vi "NanotecSMCPD.halt axis.vi"(0 "i ref in":refnum<vi>, 1 "axis":i32, 2 "ManuelStop":bool, 3 "ms timeout (10000)":i32=10000, 5 "error in (no error)":errorcluster) -> (14 "i ref out":refnum<vi>, 17 "timed out":bool, 19 "error out":errorcluster)   [LabVIEW 2014, in "NanotecSMCPD.lvlib"]
doc: "Abruptly stops the ongoing movement of the specified axis, possible loss of steps."
uses:
  NanotecSMCPD.lvlib
  CSCore/CSSystem/CoreDefs/CoreDefs.error_type.ctl
  CSCore/CSSystem/CoreDefs/CoreDefs.error_severity.ctl
  CSCore/CSApplicationBaseClasses/MotorBase/MotorBase.statusType.ctl
  CSCore/CSApplicationBaseClasses/MotorBase/MotorBase.directionType.ctl
  CSCore/CSApplicationBaseClasses/MotorBase/MotorBase.serviceType.ctl
  CSlibraries/UtilityLib/UtilityLib.valueStatus.ctl
  CSCore/CSApplicationBaseClasses/DeviceBase/DeviceBase.lvlib
  CSCore/CSSystem/CoreLib/CoreLib.lvlib
  CSCore/CSApplicationBaseClasses/MotorBase/MotorBase.lvlib
  CSlibraries/UtilityLib/UtilityLib.lvlib
  CSinstr.lib/NanotecSMCPD/NanotecSMCPDDriver.lvlib
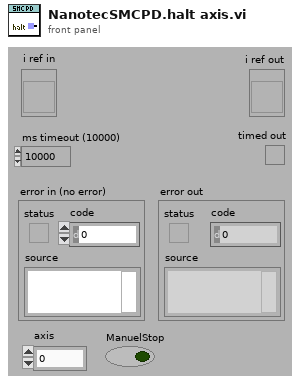
[diagram p1: front panel]
types:
  T1 = typedef "CoreDefs.error_severity.ctl" = enum16{"undefined", "information", "warning", "error", "fatal"}
  T2 = typedef "CoreDefs.error_type.ctl" = enum16{"no error", "can't load process", "can't unload process", "process does not exist", "can't install process", "can't remove process", "unknown function", "time out", "can't execute function", "duplicate queue name", "super not found", "caller queue invalid", "can't ping process", "unknown error", "VISA Error", "VISA timeout", "GPIB timeout", "GPIB error", "communication error", "data type mismatch", "can't read data from OPC server", "can't write data to OPC server", "OET error", "function not implemented", "process already exists", "invalid Shared Variable name", "error writing Shared Variable", "error reading Shared Variable", "invalid client name", "corrupt database", "unknown class", "call not authorized", "parameter out of range", "OET timeout: can't get data to modify", "invalid queue name", "requested operation incompatible with current state", "event undefined", "event disabled", "state undefined", "caller is not a friend", "EventBuilder: bad eventID", "EventBuilder: no DAQ devices", "a thread must not stop itself", "UNUSED ELEMENT4", "DiscArchiver: eventData incomplete", "DiscArchiver: eventData does not belong to run", "DiscArchiver: can't open file", "DiscArchiver: can't write to file", "DiscArchiver: available disc space low", "can't acquire semaphore", "error reading data from database", "notifier object is not existing", "can't register process", "can't unregister process", "illegal event type", "object disabled", "object already exists", "can't change state", "Instrument not found", "no connection to remote node", "invalid reference", "N/A", "UNUSED ELEMENT 1", "element not found", "illegal TCP/IP connection detected", "object does not exist", "invalid access ID", "unknown CS system", "invalid privilige", "unsupported data type", "unsupported server type", "IO server already exists", "Shared Variable already exists"}
  T3 = typedef "MotorBase.lvlib/MotorBase.serviceType.ctl" = enum16{"onOff", "startVelocity", "stopVelocity", "acceleration", "rangeMin", "rangeMax", "status", "position"}
  T4 = typedef "MotorBase.lvlib/MotorBase.directionType.ctl" = enum16{"unknown", "update actual value", "update nominal value", "update both"}
  T5 = typedef "UtilityLib.lvlib/UtilityLib.valueStatus.ctl" = enum16{"no info available", "stand by/off", "on", "warning", "alarm/malfunction", "not implemented", "user action required", "important information", "system default", "control default", "indicator default", "button default"}
  T6 = typedef "MotorBase.lvlib/MotorBase.statusType.ctl" = u32
  T7 = typedef "NanotecSMCPD.lvlib/NanotecSMCPD.i attribute.ctl" = cluster{"referencing":bool[], "stop":bool[], "AutoHalt ID":i32, "MethodQueue":refnum<queue>, "Referenced1Time?":bool[], "LastCommand ID":i32}
  T8 = typedef "MotorBase.lvlib/MotorBase.i attribute.ctl" = cluster{"defaultAxisIndex":i32, "logicalName":string[], "nOfAxes":i32, "physicalName":string[], "scaling":dbl[], "units":string[], "defaulAxisIndexID":i32, "logicalNameID":i32, "nOfAxesID":i32, "physicalNameID":i32, "unitID":i32, "actValues":T9, "nomValues":T9}
  T9 = typedef "MotorBase.lvlib/MotorBase.parameters.ctl" = cluster{"services":cluster{"onOff":bool[], "startVelocity":dbl[], "stopVelocity":dbl[], "acceleration":dbl[], "rangeMin":dbl[], "rangeMax":dbl[], "status":T6[], "position":dbl[]}, "serviceIDs":cluster{"onOffID":i32, "startVelocityID":i32, "stopVelocityID":i32, "accelerationID":i32, "rangeMinID":i32, "rangeMaxID":i32, "statusID":i32, "positionID":i32}}
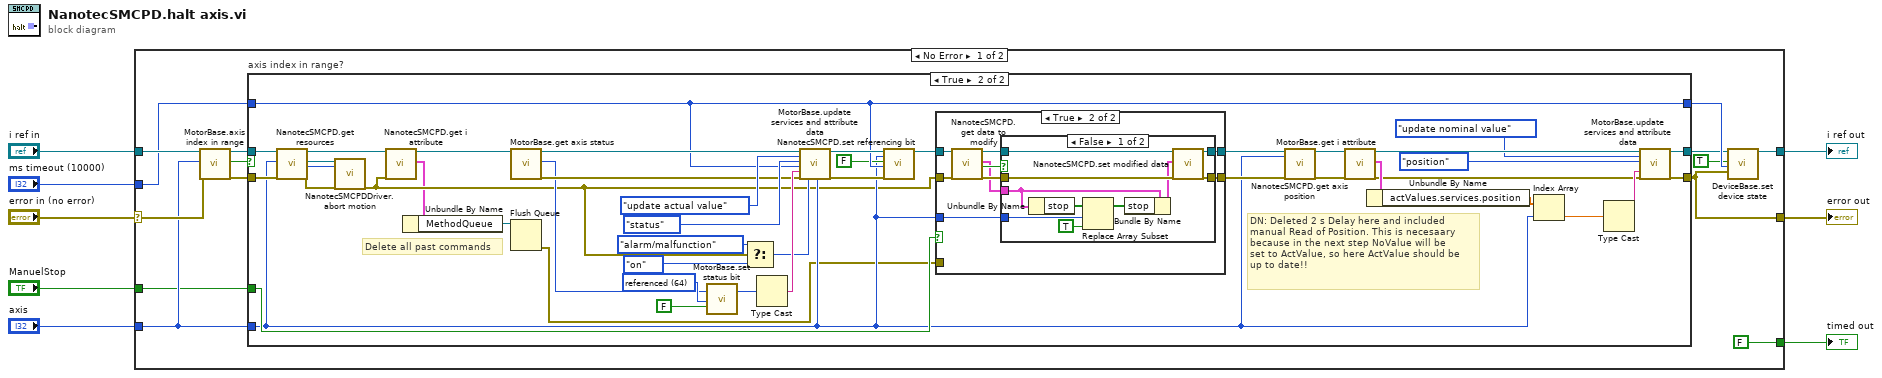
[diagram p0: block diagram]
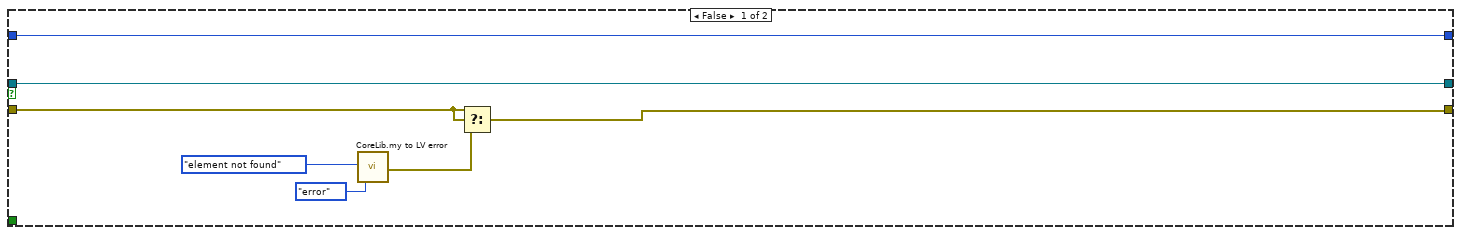
[diagram p2: hidden frame]
diagram:
  n1 = case shown="No Error" "error in (no error)" {
    selector: "error in (no error)" -> [w15 w97]
    tunnel: "ms timeout (10000)" -> [w12 _]
    tunnel: "i ref in" -> [w16 w98]
    tunnel: [w14 w97] -> w5
    tunnel: "axis" -> [w13 _]
    tunnel: [w11 w98] -> w3
    tunnel: [FALSE _] -> w2
    tunnel: "ManuelStop" -> [w9 _]
    frame No Error {
      n2 = call "MotorBase.axis index in range.vi"("i ref in"=w16, "axisIndex"=w13, "error in (no error)"=w15) -> ("i ref out"=w20:refnum<vi>, "in range"=w19:bool, "error out"=w21:errorcluster)  [unwired: 14 in]
      n3 = case "axis index in range?" shown="True" w19 {
        tunnel: [w29 w41] -> w18
        tunnel: [w26 w42] -> w14
        tunnel: w12 -> [w23 w54]
        tunnel: w13 -> [_ w36]
        tunnel: w20 -> [w29 w68]
        tunnel: w21 -> [w27 w67]
        tunnel: [w23 w54] -> w22
        tunnel: w9 -> [_ w52]
        frame False {
          n4 = call "CoreLib.my to LV error.vi"("ErrorTypes"=CoreDefs.error_type."element not found", "severityLevel"=CoreDefs.error_severity."error") -> ("myErrorCluster"=w25:errorcluster)  [unwired: 16 in, 1 out]
          n5 = Select(t=w27, s=w27, f=w25) -> (s? t:f=w26:errorcluster)
        }
        frame True {
          w64 = T6 64 items=["motorEnabled"=1, "negativeLimitSwitchActive"=2, "positiveLimitSwitchActive"=4, "limitSwitchesEnabled"=8, "limitSwitchesAreNormallyClosed"=16, "reseved1"=32, "referenced"=64, "inPosition"=128, "reserved2"=256, "reserved3"=512, "reserved4"=1024, "reserved5"=2048, "error"=4096, "reserved6"=8192, "reserved7"=16384, "reserved8"=32768, "user defined1"=65536, "user defined2"=131072, "user defined3"=262144, "user defined4"=524288, "user defined5"=1048576, "user defined6"=2097152, "user defined7"=4194304, "user defined8"=8388608, "user defined9"=16777216, "user defined10"=33554432, "user defined11"=67108864, "user defined12"=134217728, "user defined13"=268435456, "user defined14"=536870912, "user defined15"=1073741824, "user defined16"=2147483648] ("service")
          # "Delete all past commands"
          # "DN: Deleted 2 s Delay here and included\nmanual Read of Position. This is necesaary\nbecause in the next step NoValue will be\nset to ActValue, so here ActValue should be\nup to date!!"
          n6 = call "NanotecSMCPD.get resources.vi"("i ref in"=w68, "axisNumber"=w36, "error in (no error)"=w67) -> ("i ref out"=w34:refnum<vi>, "VISA resource"=w59:refnum<visa-resource-name>, "address"=w58:i32, "error out"=w66:errorcluster)  [unwired: 13 in]
          n7 = call "NanotecSMCPDDriver.abort motion.vi"("VISA resource name"=w59, "contollerID"=w58, "error in (no error)"=w66) -> ("error out"=w33:errorcluster)  [unwired: 14 in, 2 out]
          n8 = call "NanotecSMCPD.get i attribute.vi"("i ref in"=w34, "error in (no error)"=w33) -> ("i ref out"=w35:refnum<vi>, "i attribute"=w32:T7)  [unwired: 15 in, 1 out]
          n9 = Unbundle By Name(w32) -> ("MethodQueue"=w31:refnum<queue>)
          n10 = call "MotorBase.get axis status.vi"("i ref in"=w35) -> ("i ref out"=w70:refnum<vi>, "status"=w57:T6, "error out"=w69:errorcluster)  [unwired: 16 in]
          n11 = Flush Queue(queue=w31) -> (error out=w30:errorcluster)  [unwired: 1 in, 2 out]
          n12 = call "MotorBase.set status bit.vi"("status"=w57, "statusBit"=w64, "setBit"=FALSE) -> ("status out"=w65:T6)  [unwired: 16 in]
          n13 = Select(t=UtilityLib.valueStatus."alarm/malfunction", s=w33, f=UtilityLib.valueStatus."on" ("quality")) -> (s? t:f=w60:T5)
          n14 = Type Cast(x=w65) -> (*(type *) &x=w73:string)  [unwired: 1 in]
          n15 = call "MotorBase.update services and attribute data.vi"("i ref in"=w70, "direction"=MotorBase.directionType."update actual value", "service"=MotorBase.serviceType."status", "ms timeout (10000)"=w54, "value"=w73, "error in (no error)"=w69, "quality"=w60, "axisNumber"=w36) -> ("i ref out"=w56:refnum<vi>, "error out"=w55:errorcluster)  [unwired: 9 in, 1 out]
          n16 = call "NanotecSMCPD.set referencing bit.vi"("i ref in"=w56, "axis"=w36, "isReferencing?"=FALSE ("referencing?"), "ms timeout (10000)"=w54, "error in (no error)"=w55) -> ("i ref out"=w51:refnum<vi>)  [unwired: 12 in, 2 out]
          n17 = case shown="True" w52 {
            tunnel: w51 -> [w75 w84]
            tunnel: w33 -> [w74 w83]
            tunnel: [w75 w78] -> w40
            tunnel: [w74 w77] -> w38
            tunnel: w36 -> [_ w76]
            tunnel: w30 -> [_ _]
            frame False {
            }
            frame True {
              n18 = call "NanotecSMCPD.get data to modify.vi"("i ref in"=w84, "error in (no error)"=w83) -> ("i ref out"=w81:refnum<vi>, "i attribute"=w79:T7, "timed out"=w82:bool, "error out"=w80:errorcluster)  [unwired: 14 in]
              n19 = case shown="False" w82 {
                tunnel: w81 -> [w94 w96]
                tunnel: w80 -> [w91 w95]
                tunnel: w79 -> [w89 _]
                tunnel: [w93 w96] -> w78
                tunnel: [w92 w95] -> w77
                tunnel: w76 -> [w85 _]
                frame False {
                  n20 = Unbundle By Name(w89) -> ("stop"=w88:bool[])
                  n21 = Replace Array Subset(array=w88, new element=TRUE ("new element/subarray"), index=w85) -> (w87:bool[])
                  n22 = Bundle By Name(cluster=w89, "stop"=w87) -> (w90:T7)
                  n23 = call "NanotecSMCPD.set modified data.vi"("i ref in"=w94, "i attribute"=w90, "error in (no error)"=w91) -> ("i ref out"=w93:refnum<vi>, "error out"=w92:errorcluster)  [unwired: 15 in]
                }
                frame True {
                }
              }
            }
          }
          n24 = call "NanotecSMCPD.get axis position.vi"("i ref in"=w40, "axis"=w36, "error in (no error)"=w38) -> ("i ref out"=w39:refnum<vi>, "error out"=w37:errorcluster)  [unwired: 13 in, 2 out]
          n25 = call "MotorBase.get i attribute.vi"("i ref in"=w39, "error in (no error)"=w37) -> ("i ref out"=w50:refnum<vi>, "i attribute"=w47:T8, "error out"=w43:errorcluster)  [unwired: 15 in]
          n26 = Unbundle By Name(w47) -> ("actValues.services.position"=w45:dbl[])
          n27 = Index Array(array=w45, index=w36) -> (element=w44:dbl)
          n28 = Type Cast(x=w44) -> (*(type *) &x=w46:string)  [unwired: 1 in]
          n29 = call "MotorBase.update services and attribute data.vi"("i ref in"=w50, "direction"=MotorBase.directionType."update nominal value", "service"=MotorBase.serviceType."position", "value"=w46, "error in (no error)"=w43) -> ("i ref out"=w41:refnum<vi>, "error out"=w42:errorcluster)  [unwired: 12 in, 1 out]
        }
      }
      n30 = call "DeviceBase.set device state.vi"("i ref in"=w18, "implicit"=TRUE, "ms timeout (10000)"=w22, "device error"=w14) -> ("i ref out"=w11:refnum<vi>)  [unwired: 13 in, 2 out]
    }
    frame Error {
    }
  }
  "error out" <- w5
  "i ref out" <- w3
  "timed out" <- w2
